vi "upload.tdms_core.vi"(4 "Properties":map{string, string}(c390), 5 "Description":string, 7 "Name":string, 8 "error in":errorcluster, 9 "timeout (ms)":i32=300000, 10 "File Path":path, 11 "Nominal Client in":refnum<class "Nominal Client.lvclass">) -> (0 "error out":errorcluster, 2 "datasetRID":string, 3 "Nominal Client out":refnum<class "Nominal Client.lvclass">)   [LabVIEW 2020, in "Nominal Client.lvclass"]
doc: "Uploads a file to S3\nIngests video with common settings:\n - No TimeManifest (uses Start Timestamp and a scale factor of 1.\nNew Target: Name based on path name and timestamp"
uses:
  Nominal Client.lvclass
  datasources/dataset/dataset.lvclass
  nominal types/channelConfig/channelConfig.lvclass
  datasources/s3/s3.lvclass
  C:/sw/labview-client/lv_src/datasources/source/source.lvclass
  Nominal Client.lvclass/Nominal Client.ctl
  C:/sw/labview-client/lv_src/datasources/payload/payload.lvclass
  C:/sw/labview-client/lv_src/datasources/s3/s3.lvclass
  datasources/target/target.lvclass
  datasources/source/source.lvclass
  datasources/target/create_new.vi
  datasources/source/create_s3.vi
  ingest_csv.vi
  timestampMetadata/timestampMetadata.lvclass
  ts.epochOfTimeUnit/build.epoch.vi
  ts.epochOfTimeUnit/ts.epochOfTimeUnit.lvclass
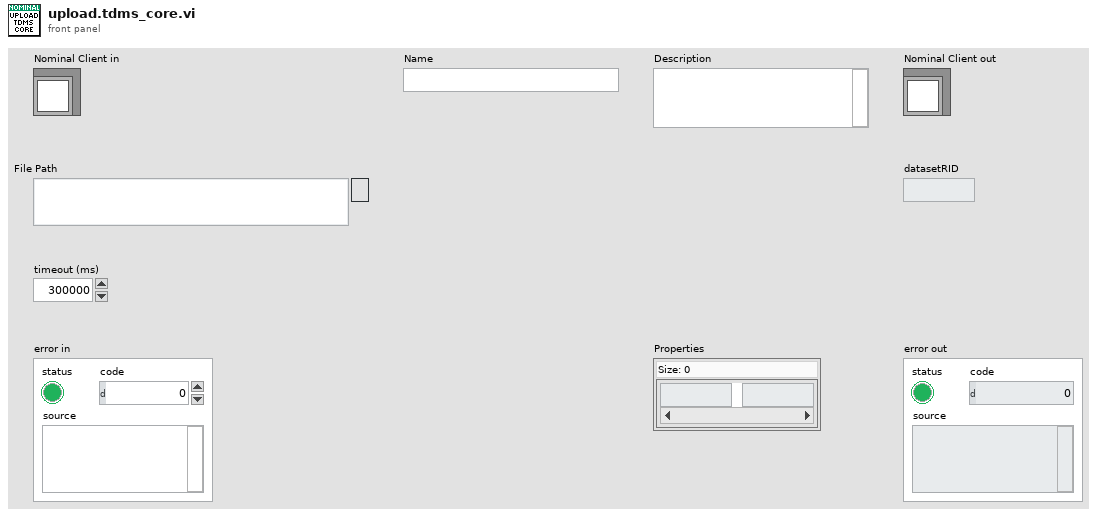
[diagram p1: front panel]
types:
  T1 = enum16{"DAYS", "HOURS", "MINUTES", "SECONDS", "MILLISECONDS", "MICROSECONDS", "NANOSECONDS", "PICOSECONDS"}
  T2 = cluster{"dataset":refnum<class "dataset.lvclass">, "channelConfig":refnum<class "channelConfig.lvclass">}
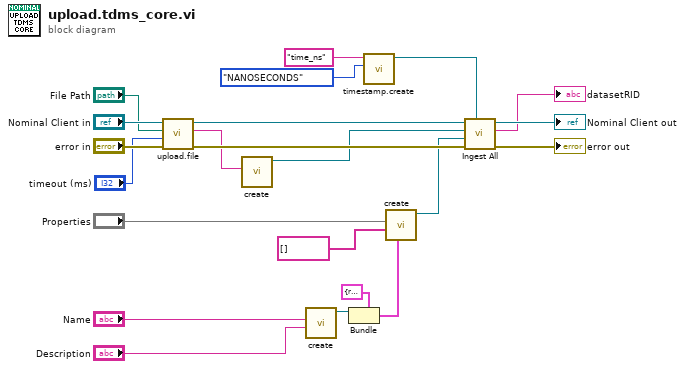
[diagram p0: block diagram]
diagram:
  n1 = call "upload.file.vi"("error in"="error in", "timeout (ms)"="timeout (ms)", "File"="File Path", "Nominal Client in"="Nominal Client in") -> ("error out"=w21:errorcluster, "Path to S3 File"=w19:string, "Nominal Client out"=w22:refnum<class "Nominal Client.lvclass">)  [unwired: 5 in]
  n2 = call-poly "create.vi"("Path"=w19) -> ("source"=w18:refnum<class "s3.lvclass">)  [unwired: 10 in]
  n3 = call "create.vi"("Description"="Description", "Name"="Name") -> ("dataset"=w17:refnum<class "dataset.lvclass">)  [unwired: 9 in]
  n4 = Bundle(cluster=T2 {"dataset"=refnum, "channelConfig"=refnum} ("Optional"), "dataset"=w17) -> (w16:T2)  [unwired: 1 in]
  n5 = call-poly "timestamp.create.vi"("Time Unit"=T1."NANOSECONDS", "Time Series Name"="time_ns") -> ("Timestamp Metadata"=w5:refnum<class "timestampMetadata.lvclass">)  [unwired: 9 in]
  n6 = call-poly "create.vi"("Optional"=w16, "Labels"=string[] [], "Properties"="Properties") -> ("New Target"=w20:refnum<class "target.lvclass">)  [unwired: 8 in]
  n7 = call-poly "Ingest All.vi"("timestampMetadata"=w5, "error in"=w21, "Target"=w20, "Source"=w18, "Nominal Client in"=w22) -> ("error out"=→"error out":errorcluster, "datasetRid"=→"datasetRID":string, "Nominal Client out"=→"Nominal Client out":refnum<class "Nominal Client.lvclass">)  [unwired: 2 in, 2 out]
